vi "replaceElement.vi"(7 "replaceElementIn":string="/child/son", 8 "error in (no error)":errorcluster, 9 "replaceWithValue":string="Dr C", 10 "replacementElementName":string="one", 11 "SettingsManager in":refnum<class "SettingsManager.lvclass">) -> (0 "error out":errorcluster, 3 "SettingsManager out":refnum<class "SettingsManager.lvclass">)   [LabVIEW 2011, in "Tools.lvlib" / "Settings.lvlib" / "SettingsManager.lvclass"]
uses:
  SettingsManager.lvclass
  SettingsManager.lvclass/SettingsManager.ctl
  xmlNode/xmlNode.lvclass
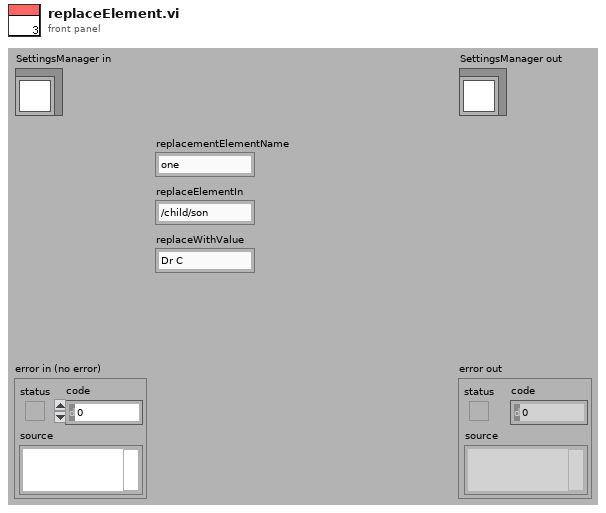
[diagram p1: front panel]
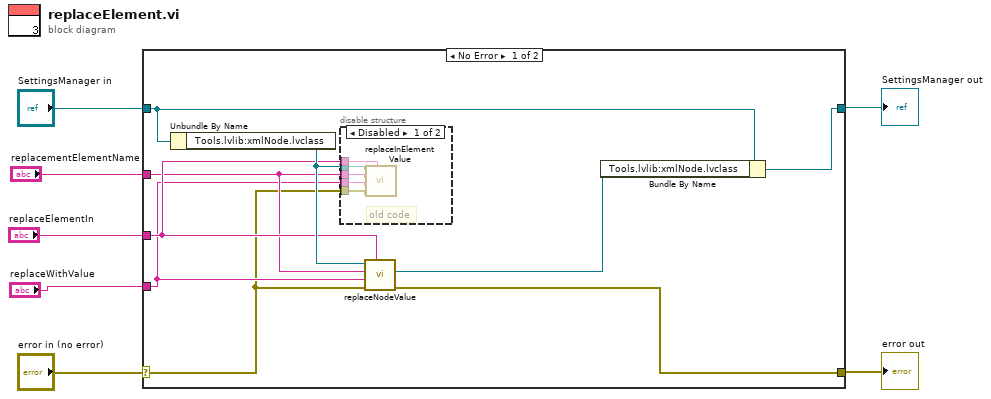
[diagram p0: block diagram]
diagram:
  n1 = case shown="No Error" "error in (no error)" {
    selector: "error in (no error)" -> [w9 w23]
    tunnel: [w8 w23] -> w6
    tunnel: [w15 w22] -> w4
    tunnel: "SettingsManager in" -> [w16 w22]
    tunnel: "replaceElementIn" -> [w13 _]
    tunnel: "replacementElementName" -> [w12 _]
    tunnel: "replaceWithValue" -> [w11 _]
    frame No Error {
      n2 = Unbundle By Name(w16) -> ("Tools.lvlib:xmlNode.lvclass"=w14:refnum<class "xmlNode.lvclass">)
      n3 = disable-structure shown="Disabled" {
        disable-tunnel: w14 -> [w21 _]
        disable-tunnel: w13 -> [w20 _]
        disable-tunnel: w12 -> [w19 _]
        disable-tunnel: w11 -> [w18 _]
        disable-tunnel: w9 -> [w17 _]
        frame Disabled {
          # "old code"
          n4 = call-dynamic "replaceInElementValue.vi"("replaceElementIn"=w20, "error in (no error)"=w17, "replaceWithValue"=w18, "replacementElementName"=w19, "xmlNode in"=w21) -> ()  [unwired: 4 in, 3 out]
        }
        frame Enabled {
        }
      }
      n5 = call "replaceNodeValue.vi"("searchInElement"=w13, "error in (no error)"=w9, "replaceWith"=w11, "replaceElement"=w12, "xmlNode in"=w14) -> ("error out"=w8:errorcluster, "xmlNodeReplacement"=w10:refnum<class "xmlNode.lvclass">)  [unwired: 4 in, 1 out]
      n6 = Bundle By Name(cluster=w16, "Tools.lvlib:xmlNode.lvclass"=w10) -> (w15:refnum<class "SettingsManager.lvclass">)
    }
    frame Error {
    }
  }
  "error out" <- w6
  "SettingsManager out" <- w4
